vi "process_main.vi"(7 "FGV_mods":enum16{"Init", "Exec", "End"}(ring), 8 "Error In":errorcluster, 11 "DataIn":variant) -> (0 "Error Out":errorcluster, 3 "DataOut":variant)   [LabVIEW 2016]
uses:
  process_data.ctl
  CurrentMeter/CM_data.ctl
  CurrentMeter/CM_SerialNumber.ctl
  StrainGauge/SG_data.ctl
  MainFGV/MainFGV_data.ctl
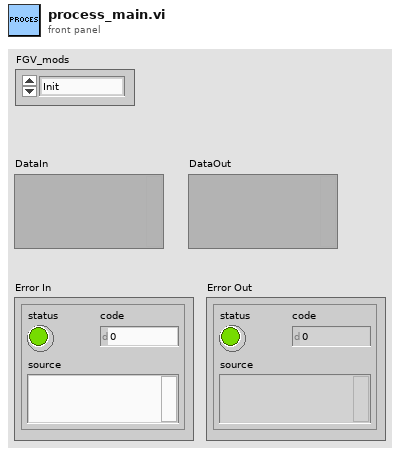
[diagram p1: front panel]
types:
  T1 = typedef "MainFGV_data.ctl" = cluster{"TestDir":path, "TestName":string, "CM_data":T2[], "SG_data":T4[], "Simulation":bool, "task":refnum<k21>, "data_file":refnum<file>, "data_bursts":refnum<file>, "data_log":refnum<file>}
  T2 = typedef "CM_data.ctl" = cluster{"Serial":T3, "Coordenada X":dbl, "Coordenada Y":dbl, "ID":string, "active":bool}
  T3 = typedef "CM_SerialNumber.ctl" = enum16{"274124", "274125", "274126", "274127", "274128"}
  T4 = typedef "SG_data.ctl" = cluster{"ID":string, "Sensibilidade":dbl, "Descrição":string, "active":bool}
  T5 = typedef "process_data.ctl" = cluster{"CM_data":T2[], "SG_data":T4[]}
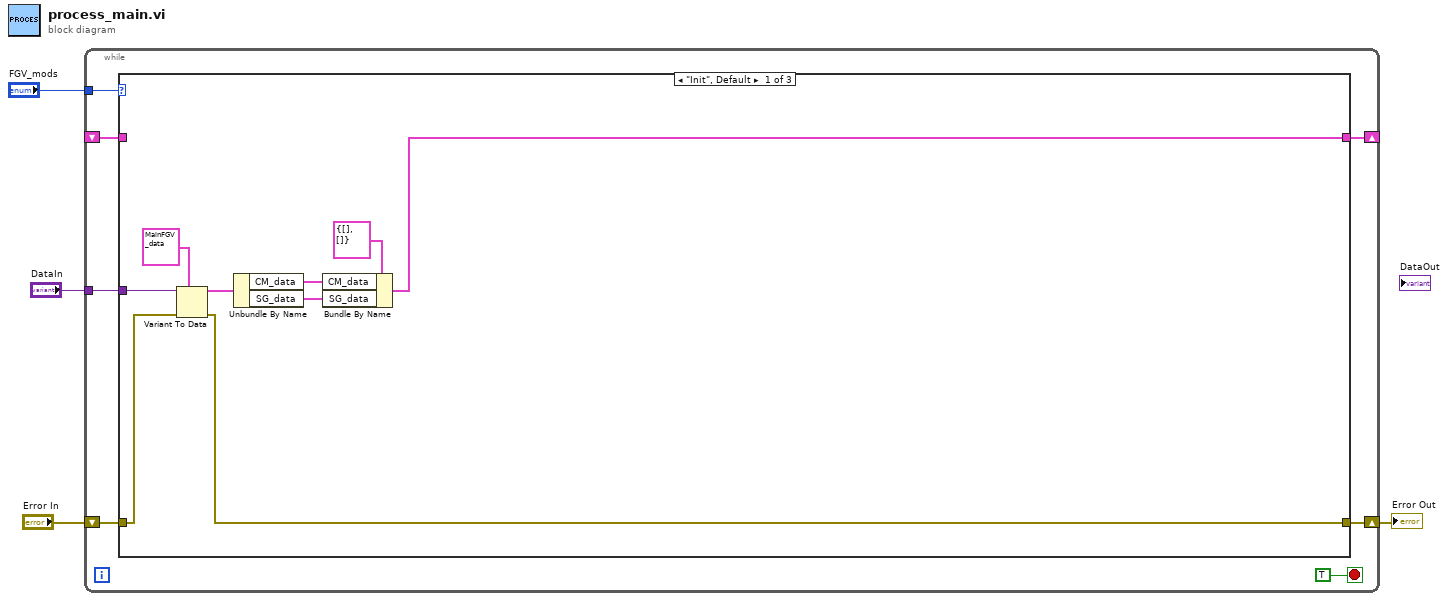
[diagram p0: block diagram]
diagram:
  n1 = while {
    tunnel: "DataIn" -> [w10]
    tunnel: "FGV_mods" -> [w9]
    shift-right: [w8] -> _
    shift-left: _ -> [w7]
    shift-right: [w5] -> w1
    shift-left: "Error In" -> [w6]
    stop <- TRUE stop-if-true
    n2 = case shown="\"Init\", Default" w9 {
      tunnel: w10 -> [w20 _ _]
      tunnel: [w13 w22 w24] -> w8
      tunnel: w7 -> [_ w22 w24]
      tunnel: w6 -> [w19 w21 w23]
      tunnel: [w12 w21 w23] -> w5
      frame "Init", Default {
        n3 = Variant To Data(error in=w19, type=T1 {"TestDir"=path "", "TestName"="", "CM_data"=[], "SG_data"=[], "Simulation"=FALSE, "task"="", "data_file"=refnum, "data_bursts"=refnum, "data_log"=refnum} ("MainFGV_data"), Variant=w20) -> (data=w17:T1, error out=w12:errorcluster)
        n4 = Unbundle By Name(w17) -> ("CM_data"=w15:T2[], "SG_data"=w14:T4[])
        n5 = Bundle By Name(cluster=T5 {"CM_data"=[], "SG_data"=[]} ("process_data"), "CM_data"=w15, "SG_data"=w14) -> (w13:T5)
      }
      frame "Exec" {
      }
      frame "End" {
      }
    }
  }
  "Error Out" <- w1
